vi "Decode Single (ARGB Flat).vi"(8 "error in (no error)":errorcluster, 9 "Detection":T1, 10 "ARGB Image in":T3, 11 "QR Code Detector in":refnum<class "QR Code Detector.lvclass">) -> (0 "error out":errorcluster, 2 "Data":string, 3 "QR Code Detector":refnum<class "QR Code Detector.lvclass">)   [LabVIEW 2020, in "feature_detection.lvlib" / "QR Code Detector.lvclass"]
doc: "Decode a single QR Code at the location specified."
uses:
  QR Code Detector.lvclass
  image/ARGB Image.ctl
  common/Image Points Quad (Float).ctl
  common/Image Point (Float).ctl
  QR Code Detector.lvclass/QR Code Detector.ctl
  94f8c690-e24c-46ee-a000-65550b546d0d.vi
  <vilib>/Utility/error.llb/Error Cluster From Error Code.vi
  image/image.lvlib
  common/common.lvlib
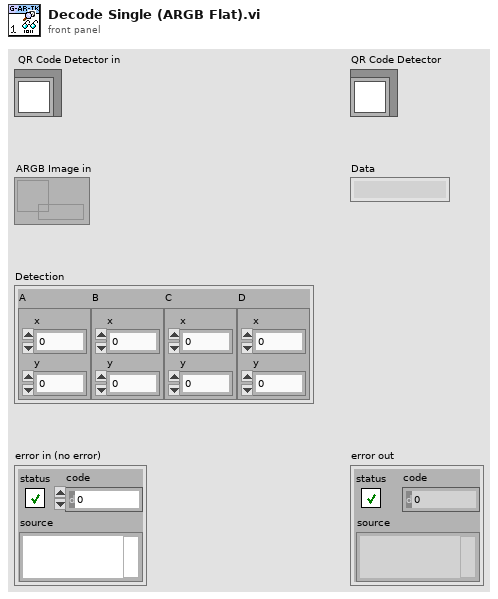
[diagram p1: front panel]
types:
  T1 = typedef "common.lvlib/Image Points Quad (Float).ctl" = cluster{"A":T2, "B":T2, "C":T2, "D":T2}
  T2 = typedef "common.lvlib/Image Point (Float).ctl" = cluster{"x":dbl, "y":dbl}
  T3 = typedef "image.lvlib/ARGB Image.ctl" = refnum<data-value>
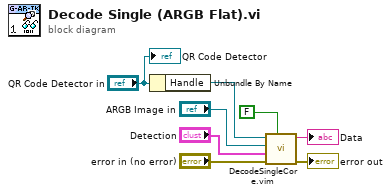
[diagram p0: block diagram]
diagram:
  n1 = Unbundle By Name("QR Code Detector in") -> ("Handle"=w6:refnum<data-value>)
  n2 = call "DecodeSingleCore.vim"("is curved?"=FALSE, "error in (no error)"="error in (no error)", "Detection"="Detection", "Greyscale Image"="ARGB Image in", "Handle"=w6) -> ("error out"=→"error out":errorcluster, "Info"=→"Data":string)  [unwired: 5 in]
  "QR Code Detector" <- "QR Code Detector in"
